vi "LoadBufferForMultiListBoxAndFormat.vi"(6 "MCListbox Refnum":refnum<vi>, 7 "configuration in":T2, 8 "error in (no error)":errorcluster, 9 "channel names in":string[](array[string]), 10 "group names in":string[](array[string]), 11 "TDMS descriptor array":T1(array[cluster])) -> (0 "error out":errorcluster, 3 "TDMS descriptor array out":T1(array[cluster]))   [LabVIEW 2015]
uses:
  <vilib>/Utility/tdmsutil.llb/fileViewerConfigData.ctl
panel:
  out "tdms file out":refnum<k34>
  in  "tdms file in":refnum<k34>
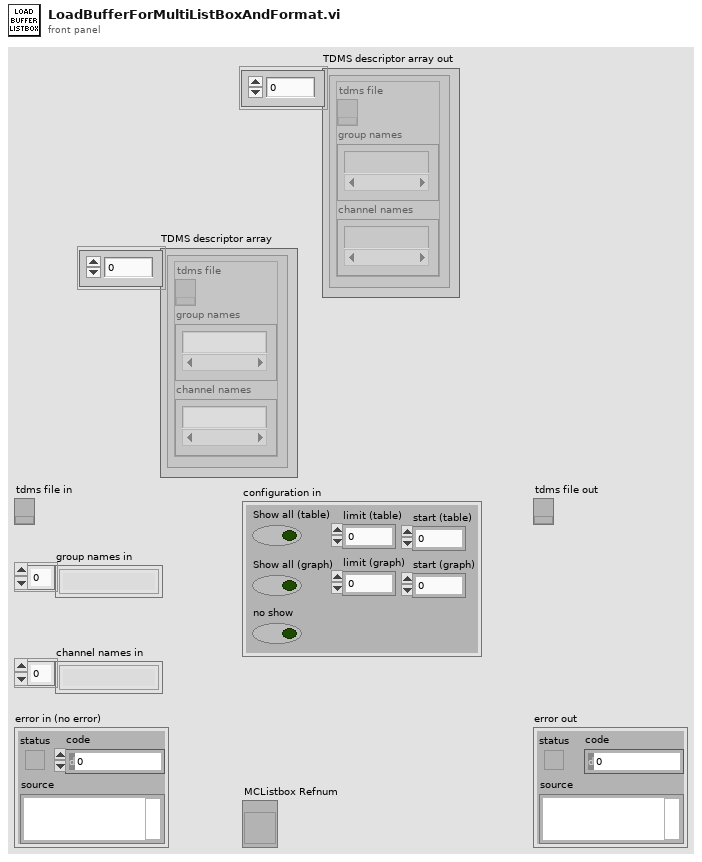
[diagram p1: front panel]
types:
  T1 = cluster{"tdms file ":refnum<k34>, "group names":string[], "channel names":string[]}[]
  T2 = typedef "fileViewerConfigData.ctl" = cluster{"Show all (table)":bool, "Show all (graph)":bool, "limit (table)":u64, "limit (graph)":u64, "no show":bool, "start (table)":u64, "start (graph)":u64}
  T3 = cluster{"tdms file ":refnum<k34>, "group names":string[], "channel names":string[]}
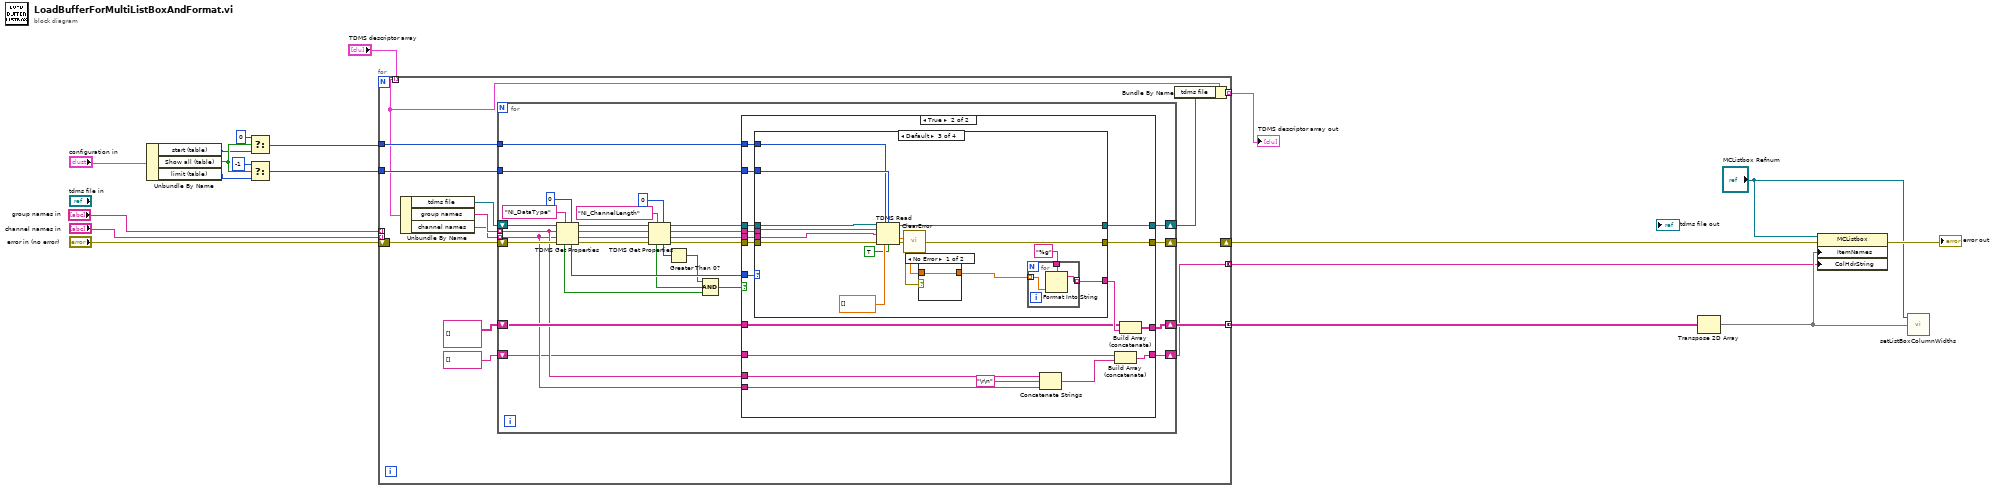
[diagram p0: block diagram]
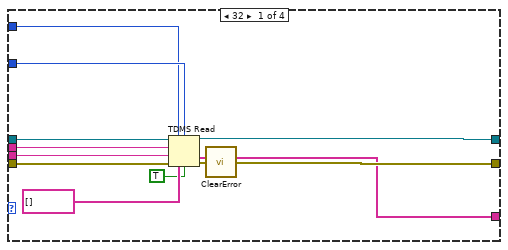
[diagram p3: hidden frame]
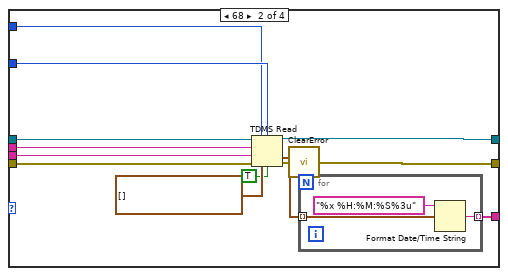
[diagram p4: hidden frame]
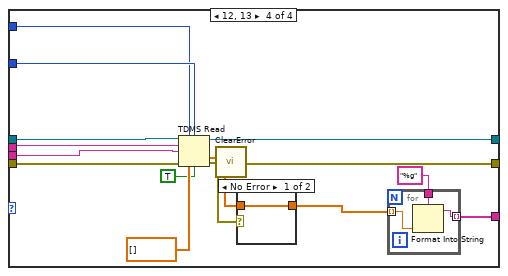
[diagram p6: hidden frame]
diagram:
  n1 = Unbundle By Name("configuration in") -> ("start (table)"=w14:u64, "Show all (table)"=w15:bool, "limit (table)"=w16:u64)
  n2 = Select(t=u64 0, s=w15, f=w14) -> (s? t:f=w17:u64)
  n3 = Select(t=i64 -1 ("count (-1: all)"), s=w15, f=w16) -> (s? t:f=w18:u64)
  n4 = for {
    tunnel: w18 -> [w33]
    tunnel: w17 -> [w32]
    tunnel: "channel names in" -> [_] mode=indexing
    tunnel: "group names in" -> [_] mode=indexing
    tunnel: [w30] -> w8 mode=concatenating
    tunnel: [w27] -> w6 mode=concatenating
    shift-right: [w26] -> w5
    shift-left: "error in (no error)" -> [w31]
    tunnel: "TDMS descriptor array" -> [w22] mode=indexing
    tunnel: [w21] -> w1 mode=indexing
    n5 = Unbundle By Name(w22) -> ("tdms file"=w25:refnum<k34>, "group names"=w24:string[], "channel names"=w23:string[])
    n6 = for {
      tunnel: w23 -> [w36] mode=indexing
      shift-right: [w62] -> w26
      shift-left: w31 -> [w61]
      shift-right: [w63] -> w20
      shift-left: w25 -> [w60]
      tunnel: w24 -> [w37] mode=indexing
      tunnel: w33 -> [w56]
      tunnel: w32 -> [w55]
      shift-right: [w38] -> w30
      shift-left: string[][] [] -> [w39]
      shift-right: [w34] -> w27
      shift-left: string[] [] -> [w35]
      n7 = TDMS Get Properties(5:u16 0, 7:"NI_DataType" ("property name"), 8:w61, 9:w36, 10:w37, 11:w60) -> (0:w54:errorcluster, 1:w47:string, 2:w48:string, 3:w53:refnum<k34>, 4:w57:u16, 6:w41:bool)
      n8 = TDMS Get Properties(5:u64 0, 7:"NI_ChannelLength" ("property name"), 8:w54, 9:w47, 10:w48, 11:w53) -> (0:w52:errorcluster, 1:w51:string, 2:w50:string, 3:w49:refnum<k34>, 4:w44:u64, 6:w42:bool)
      n9 = Greater Than 0?(x=w44) -> (x > 0?=w43:bool)
      n10 = Compound Arithmetic op=AND(w43, w42, w41) -> (w40:bool)
      n11 = case shown="True" w40 {
        tunnel: [w67 w85] -> w63
        tunnel: [w66 w77] -> w62
        tunnel: w49 -> [w67 w84]
        tunnel: w52 -> [w66 w83]
        tunnel: w50 -> [_ w82]
        tunnel: w51 -> [_ w81]
        tunnel: w57 -> [_ w80]
        tunnel: w56 -> [_ w79]
        tunnel: w55 -> [_ w78]
        tunnel: w39 -> [w65 w74]
        tunnel: [w65 w75] -> w38
        tunnel: w37 -> [_ w72]
        tunnel: w36 -> [_ w68]
        tunnel: w35 -> [w64 w71]
        tunnel: [w64 w69] -> w34
        frame False {
        }
        frame True {
          n12 = case shown="Default" w80 {
            tunnel: [w91 w104 w125 w144] -> w85
            tunnel: [w92 w105 w126 w145] -> w77
            tunnel: [w90 w103 w119 w138] -> w76
            tunnel: w84 -> [w97 w110 w117 w136]
            tunnel: w83 -> [w94 w107 w114 w133]
            tunnel: w82 -> [w96 w109 w116 w135]
            tunnel: w81 -> [w95 w108 w115 w134]
            tunnel: w79 -> [w89 w101 w124 w143]
            tunnel: w78 -> [w88 w100 w123 w142]
            frame 32 {
              n13 = TDMS Read(0:w97, 1:w88, 2:w89, 5:w96, 7:w95, 11:w94, 12:string[] [], 13:TRUE ("return channels in file order? (F)")) -> (4:w91:refnum<k34>, 10:w90:string[], 15:w87:errorcluster)  [unwired: 3 out]
              n14 = call <vilib>:"ClearError.vi"("error in (no error)"=w87) -> ("error out"=w92:errorcluster)
            }
            frame 68 {
              n15 = TDMS Read(0:w110, 1:w100, 2:w101, 5:w109, 7:w108, 11:w107, 12:timestamp[] [], 13:TRUE ("return channels in file order? (F)")) -> (4:w104:refnum<k34>, 10:w102:timestamp[], 15:w99:errorcluster)  [unwired: 3 out]
              n16 = call <vilib>:"ClearError.vi"("error in (no error)"=w99) -> ("error out"=w105:errorcluster)
              n17 = for {
                tunnel: [w113] -> w103 mode=indexing
                tunnel: w102 -> [w112] mode=indexing
                n18 = Format Date/Time String(time format string (%c)="%x %H:%M:%S%3u", seconds (now)=w112) -> (date/time string=w113:string)  [unwired: 1 in]
              }
            }
            frame Default {
              n19 = TDMS Read(0:w117, 1:w123, 2:w124, 5:w116, 7:w115, 11:w114, 12:dbl[] [], 13:TRUE ("return channels in file order? (F)")) -> (4:w125:refnum<k34>, 10:w128:dbl[], 15:w122:errorcluster)  [unwired: 3 out]
              n20 = call <vilib>:"ClearError.vi"("error in (no error)"=w122) -> ("error out"=w126:errorcluster)
              n21 = case shown="No Error" w126 {
                tunnel: w128 -> [w132 _]
                tunnel: [w132 _] -> w120
                frame No Error {
                }
                frame Error {
                }
              }
              n22 = for {
                tunnel: "%g" ("format string") -> [w131]
                tunnel: w120 -> [w130] mode=indexing
                tunnel: [w129] -> w119 mode=indexing
                n23 = Format Into String(format string=w131, w130) -> (resulting string=w129:string)  [unwired: 2 in, 1 out]
              }
            }
            frame 12, 13 {
              n24 = TDMS Read(0:w136, 1:w142, 2:w143, 5:w135, 7:w134, 11:w133, 12:cdb[] [], 13:TRUE ("return channels in file order? (F)")) -> (4:w144:refnum<k34>, 10:w147:cdb[], 15:w141:errorcluster)  [unwired: 3 out]
              n25 = call <vilib>:"ClearError.vi"("error in (no error)"=w141) -> ("error out"=w145:errorcluster)
              n26 = case shown="No Error" w145 {
                tunnel: w147 -> [w151 _]
                tunnel: [w151 _] -> w139
                frame No Error {
                }
                frame Error {
                }
              }
              n27 = for {
                tunnel: "%g" ("format string") -> [w150]
                tunnel: w139 -> [w149] mode=indexing
                tunnel: [w148] -> w138 mode=indexing
                n28 = Format Into String(format string=w150, w149) -> (resulting string=w148:string)  [unwired: 2 in, 1 out]
              }
            }
          }
          n29 = Concatenate Strings(w72, "\r\n", w68) -> (w70:string)
          n30 = Build Array (concatenate)(w71, w70) -> (w69:string[])
          n31 = Build Array (concatenate)(w74, w76) -> (w75:string[][])
        }
      }
    }
    n32 = Bundle By Name(cluster=w22, "tdms file"=w20) -> (w21:T3)
  }
  "TDMS descriptor array out" <- w1
  n33 = Transpose 2D Array(2D array=w8) -> (transposed array=w7:string[][])
  n34 = property on="Property Node" class="MCListbox"(reference="MCListbox Refnum", error in=w5, "ItemNames"=w7, "ColHdrString"=w6) -> (error out=→"error out":errorcluster)  [unwired: 1 out]
  n35 = call <vilib>:"setListBoxColumnWidths.vi"("table data"=w7, "MCListbox Refnum"="MCListbox Refnum") -> ()  [unwired: 1 out]
